vi "TSM SSC DAQmx Configure Regeneration.vi"(0 "TSM DAQmx In":T1, 5 "RegenMode":i32(ring)=10097 items=["Allow Regeneration"=10097, "Do Not Allow Regeneration"=10158], 11 "error in (no error)":errorcluster) -> (4 "TSM DAQmx Out":T1, 15 "error out":errorcluster)   [LabVIEW 2020]
doc: "Specifies whether to allow NI-DAQmx to generate the same data multiple times."
uses:
  Pin Map/TSM DAQmx Multi-Task.ctl
  <vilib>/NI_TestStand_SemiconductorModule/NI_TestStand_Semiconductor_Module.lvlibp/PinMap/PinQueryContext/MultiplePinMultipleSessionQueryContext/MultiplePinMultipleSessionQueryContext.lvclass
  Pin Map/SSC DAQmx.ctl
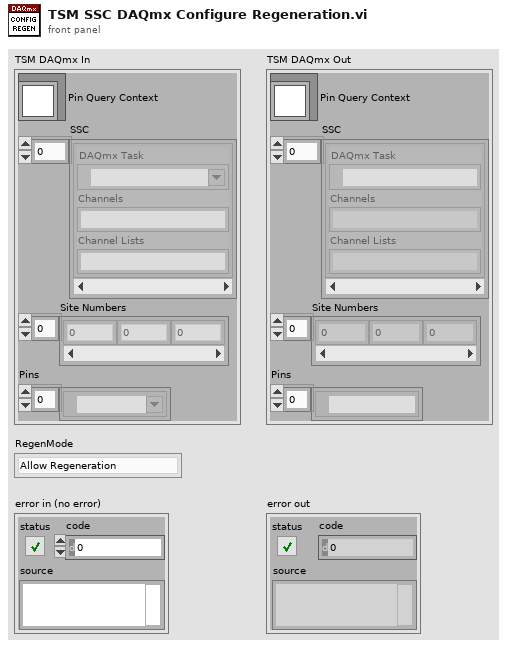
[diagram p1: front panel]
types:
  T1 = typedef "TSM DAQmx Multi-Task.ctl" = cluster{"Pin Query Context":refnum<class "MultiplePinMultipleSessionQueryContext.lvclass">, "SSC":T2[], "Site Numbers":i32[], "Pins":tag[]}
  T2 = typedef "SSC DAQmx.ctl" = cluster{"DAQmx Task ":refnum<k21>, "Channels":string, "Channel Lists":string}
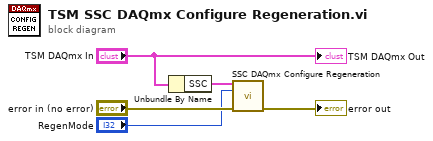
[diagram p0: block diagram]
diagram:
  n1 = Unbundle By Name("TSM DAQmx In") -> ("SSC"=w3:T2[])
  n2 = call "SSC DAQmx Configure Regeneration.vi"("DAQmx SSC in"=w3, "RegenMode"="RegenMode", "error in"="error in (no error)") -> ("error out"=→"error out":errorcluster)  [unwired: 11 in, 1 out]
  "TSM DAQmx Out" <- "TSM DAQmx In"
